vi "get_output_status.vi"(8 "error in":errorcluster, 11 "VISA resource name":refnum<visa-resource-name>="COM1") -> (0 "error out":errorcluster, 3 "VISA resource name out":refnum<visa-resource-name>)   [LabVIEW 2020]
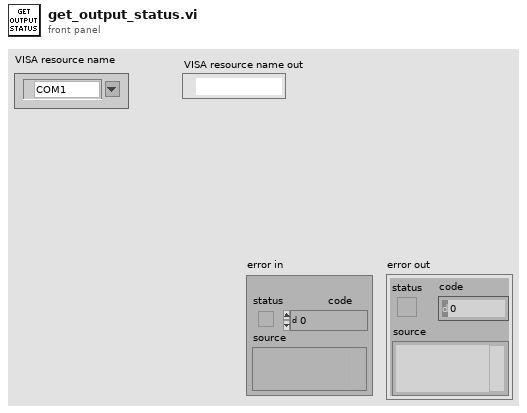
[diagram p1: front panel]
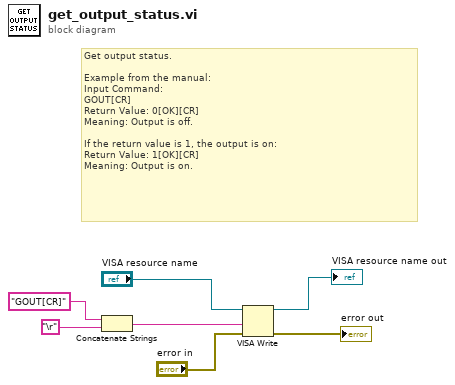
[diagram p0: block diagram]
diagram:
  # "Get output status.\n\nExample from the manual:\nInput Command:\nGOUT[CR]\nReturn Value: 0[OK][CR]\nMeaning: Output is off.\n\nIf the return value is 1, the output is on:\nReturn Value: 1[OK][CR]\nMeaning: Output is on."
  n1 = Concatenate Strings("GOUT[CR]" ("Command"), "\r") -> (w4:string)
  n2 = VISA Write(VISA resource name="VISA resource name", write buffer=w4, error in (no error)="error in") -> (VISA resource name out=→"VISA resource name out":refnum<visa-resource-name>, error out=→"error out":errorcluster)  [unwired: 1 out]
